vi "发送文件.vi"(10 "布尔":bool, 11 "VISA资源名称":refnum<visa-resource-name>) -> ()   [LabVIEW 2016]
uses:
  <vilib>/Utility/xml.llb/Read From XML File(string).vi
panel:
  out "文件大小":i64
  out "后缀名":string caption="小写文件扩展名"
  out "文件名":string
  out "错误输出":errorcluster
  out "文本信息":string
  out "进度条":u8(slide) scale=0.0..100.0
  in  "载入文件":bool
  out "提示信息":string
  in  "发送文件":bool
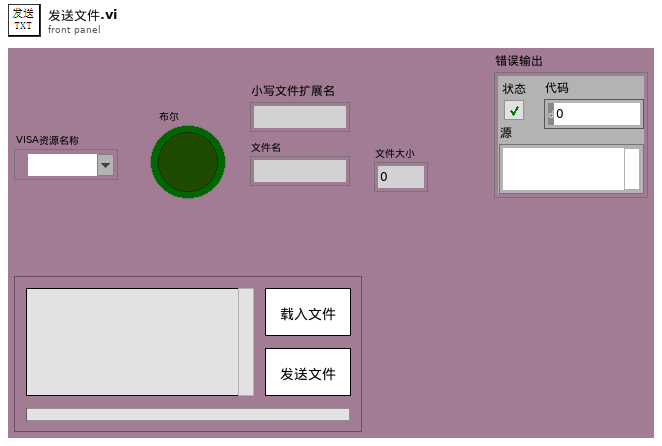
[diagram p1: front panel]
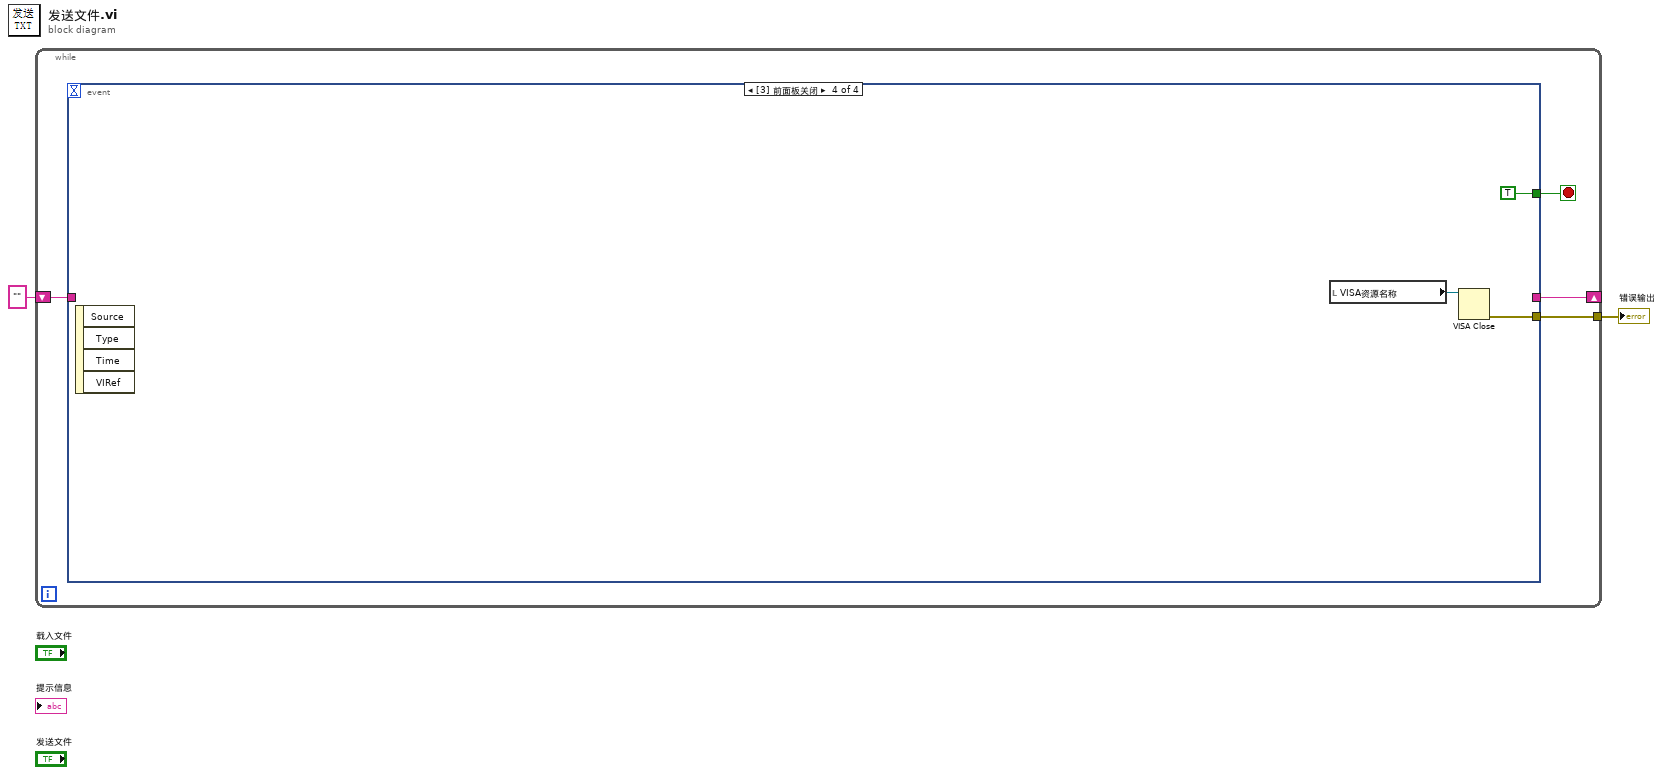
[diagram p0: block diagram]
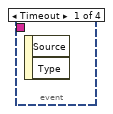
[diagram p2: hidden frame]
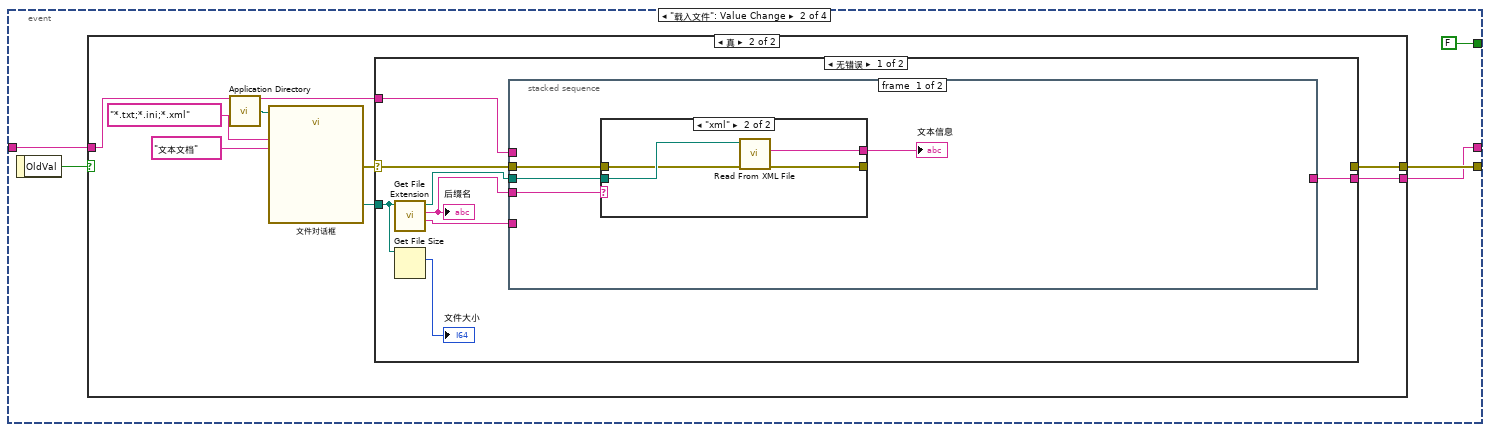
[diagram p3: hidden frame]
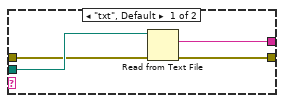
[diagram p5: hidden frame]
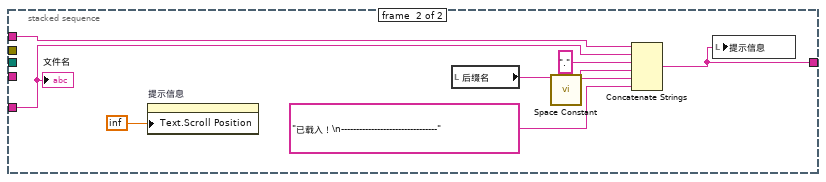
[diagram p6: hidden frame]
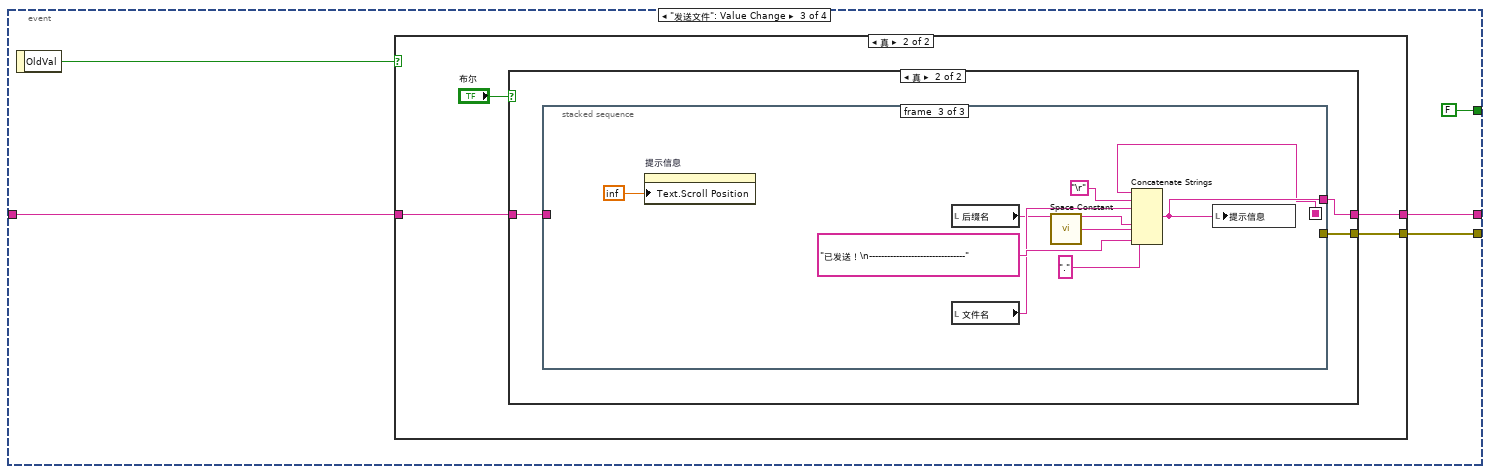
[diagram p8: hidden frame]
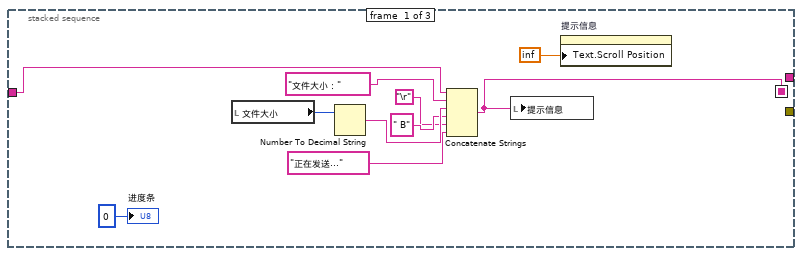
[diagram p11: hidden frame]
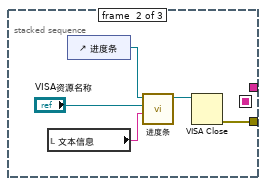
[diagram p12: hidden frame]
diagram:
  n1 = while {
    tunnel: [w5] -> w2
    shift-right: [w4] -> _
    shift-left: "" -> [w3]
    stop <- w6 stop-if-true
    n2 = event shown="[3] 前面板关闭" {
      selector: _ -> [_ _ _ _]
      dyn-events: _ -> [_ _ _ _]
      timeout: _ -> [_ _ _ _]
      tunnel: [_ FALSE FALSE TRUE] -> w6
      tunnel: [_ w9 w53 w89] -> w5
      tunnel: [_ w7 w52 _] -> w4
      tunnel: w3 -> [_ w8 w51 _]
      event Timeout {
        n3 = event-data() -> ()  [unwired: 1 in, 2 out]
      }
      event "载入文件": Value Change {
        n4 = event-data() -> ("OldVal"=w11:bool)  [unwired: 1 in]
        n5 = case shown="真" w11 {
          tunnel: [_ w15] -> w9
          tunnel: w8 -> [w12 w14]
          tunnel: [w12 w13] -> w7
          frame False {
          }
          frame True {
            n6 = call <vilib>:"Application Directory.vi"() -> ("Application Directory"=w20:path)
            n7 = call "文件对话框"("start path"=w20, "pattern (all files)"="*.txt;*.ini;*.xml", "pattern label"="文本文档") -> ("selected path"=w17:path, "error out"=w16:errorcluster)  [unwired: 9 in, 2 out]
            n8 = case shown="无错误" w16 {
              selector: w16 -> [w28 w50]
              tunnel: w17 -> [w25 _]
              tunnel: [_ w50] -> w15
              tunnel: w14 -> [w22 w49]
              tunnel: [w21 w49] -> w13
              frame No Error {
                n9 = call <vilib>:"Get File Extension.vi"("file"=w25) -> ("filename without extension"=w26:string, "lowercase file extension"=w23:string, "dup file"=w27:path)  [unwired: 6 in, 2 out]
                "后缀名" <- w23
                n10 = Get File Size(file=w25) -> (size (in bytes)=→"文件大小":i64)  [unwired: 1 in, 2 out]
                n11 = stacked-sequence {
                  tunnel: w28 -> [w30 _]
                  tunnel: w27 -> [w32 _]
                  tunnel: w23 -> [w31 _]
                  tunnel: w26 -> [_ w45]
                  tunnel: w22 -> [_ w43]
                  tunnel: [_ w42] -> w21
                  frame #0 {
                    n12 = case shown="\"xml\"" w31 {
                      tunnel: w32 -> [w36 w40]
                      tunnel: [w35 w38] -> w29
                      tunnel: [w34 w39] -> _
                      tunnel: w30 -> [w33 w37]
                      frame "txt", Default {
                        n13 = Read from Text File(file (use dialog)=w36, error in=w33) -> (text=w35:string, error out=w34:errorcluster)  [unwired: 2 in, 2 out]
                      }
                      frame "xml" {
                        n14 = call-poly <vilib>:"Read From XML File.vi"("error in (no error)"=w37, "XML File Path"=w40) -> ("error out"=w39:errorcluster, "XML Elements"=w38:string)  [unwired: 7 in, 1 out]
                      }
                    }
                    "文本信息" <- w29
                  }
                  frame #1 {
                    n15 = property on="提示信息" class="Str"("Text.Scroll Position"=inf) -> ()  [unwired: 2 in, 2 out]
                    n16 = local read "后缀名"() -> (w44:string)
                    n17 = call <vilib>:"Space Constant.vi"() -> ("String"=w47:string)
                    n18 = Concatenate Strings(w43, w45, "." ("字符串"), w44, w47, "已载入！\n--------------------------------" ("信息提示")) -> (w42:string)
                    n19 = local write "提示信息"(w42) -> ()
                    "文件名" <- w45
                  }
                }
              }
              frame Error {
              }
            }
          }
        }
      }
      event "发送文件": Value Change {
        n20 = event-data() -> ("OldVal"=w55:bool)  [unwired: 1 in]
        n21 = case shown="真" w55 {
          tunnel: [_ w59] -> w53
          tunnel: [w56 w58] -> w52
          tunnel: w51 -> [w56 w57]
          frame False {
          }
          frame True {
            n22 = case shown="真" "布尔" {
              tunnel: [_ w64] -> w59
              tunnel: [w61 w63] -> w58
              tunnel: w57 -> [w61 w62]
              frame False {
              }
              frame True {
                n23 = stacked-sequence {
                  seq-local: [w68 _ _] -> [_ _ w82]
                  tunnel: [_ w78 _] -> w64
                  tunnel: [_ _ w83] -> w63
                  tunnel: w62 -> [w67 _ _]
                  frame #0 {
                    n24 = local read "文件大小"() -> (w70:i64)
                    n25 = Number To Decimal String(number=w70) -> (decimal integer string=w73:string)  [unwired: 1 in]
                    n26 = Concatenate Strings(w67, "文件大小：" ("字符串"), w73, " B" ("字符串"), "\r", "正在发送..." ("字符串")) -> (w68:string)
                    n27 = local write "提示信息"(w68) -> ()
                    n28 = property on="提示信息" class="Str"("Text.Scroll Position"=inf) -> ()  [unwired: 2 in, 2 out]
                    "进度条" <- u8 0 ("进度条")
                  }
                  frame #1 {
                    n29 = local read "文本信息"() -> (w76:string)
                    n30 = control-ref of="进度条"() -> (w75:refnum<vi>)
                    n31 = call "进度条.vi"("文本信息"=w76, "VISA资源名称"="VISA资源名称", "Slide输入"=w75) -> ("VISA引用句柄输出"=w79:refnum<visa-resource-name>)  [unwired: 8 in]
                    n32 = VISA Close(VISA resource name=w79) -> (error out=w78:errorcluster)  [unwired: 1 in]
                  }
                  frame #2 {
                    n33 = property on="提示信息" class="Str"("Text.Scroll Position"=inf) -> ()  [unwired: 2 in, 2 out]
                    n34 = local read "后缀名"() -> (w84:string)
                    n35 = local read "文件名"() -> (w85:string)
                    n36 = call <vilib>:"Space Constant.vi"() -> ("String"=w87:string)
                    n37 = Concatenate Strings(w82, "\r", w85, "." ("字符串"), w84, w87, "已发送！\n--------------------------------" ("字符串")) -> (w83:string)
                    n38 = local write "提示信息"(w83) -> ()
                  }
                }
              }
            }
          }
        }
      }
      event Panel Close {
        n39 = event-data() -> ()  [unwired: 1 in, 4 out]
        n40 = local read "VISA资源名称"() -> (w90:refnum<visa-resource-name>)
        n41 = VISA Close(VISA resource name=w90) -> (error out=w89:errorcluster)  [unwired: 1 in]
      }
    }
  }
  "错误输出" <- w2
